vi "Search for Path.vi"(8 "error in (no error)":errorcluster, 10 "nodepath":string, 11 "Custom Device Ref":refnum<k24>) -> (0 "error out":errorcluster, 2 "BaseNodeType":refnum<k24>, 3 "Custom Device Ref":refnum<k24>)   [LabVIEW 2013, in "Control SysDef API.lvlib"]
uses:
  Control SysDef API.lvlib
  NationalInstruments.VeriStand.SystemDefinitionAPI
  NationalInstruments.VeriStand.SystemStorage
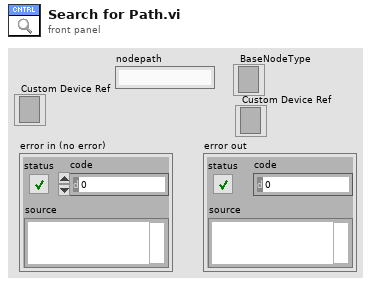
[diagram p1: front panel]
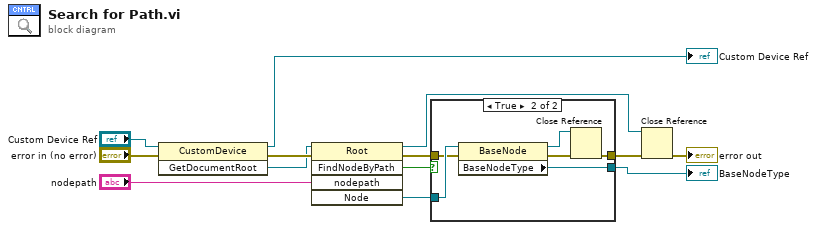
[diagram p0: block diagram]
diagram:
  n1 = invoke class="CustomDevice" method="GetDocumentRoot"(reference="Custom Device Ref", error in="error in (no error)") -> (reference out=→"Custom Device Ref":refnum<k24>, error out=w11:errorcluster, "GetDocumentRoot"=w8:refnum<k24>)  [unwired: 1 in]
  n2 = invoke class="Root" method="FindNodeByPath"(reference=w8, error in=w11, "nodepath"="nodepath") -> (reference out=w3:refnum<k24>, error out=w10:errorcluster, "FindNodeByPath"=w12:bool, "Node"=w9:refnum<k24>)  [unwired: 2 in, 1 out]
  n3 = case shown="True" w12 {
    tunnel: w9 -> [_ w20]
    tunnel: w10 -> [w14 w19]
    tunnel: [_ w18] -> w6
    tunnel: [w14 w16] -> w4
    frame False {
    }
    frame True {
      n4 = property class="BaseNode"(reference=w20, error in=w19) -> (reference out=w15:refnum<k24>, error out=w17:errorcluster, "BaseNodeType"=w18:refnum<k24>)
      n5 = Close Reference(reference=w15, error in (no error)=w17) -> (error out=w16:errorcluster)
    }
  }
  "BaseNodeType" <- w6
  n6 = Close Reference(reference=w3, error in (no error)=w4) -> (error out=→"error out":errorcluster)
